vi "Get Paths.vi"(8 "error in":errorcluster, 10 "Naming Data":refnum<class "Naming Data.lvclass">, 11 "Namer With Shared Approved File in":refnum<class "Namer With Shared Approved File.lvclass">) -> (0 "error out":errorcluster, 1 "Received Path":path, 2 "Approved Path":path, 3 "Namer With Shared Approved File out":refnum<class "Namer With Shared Approved File.lvclass">)   [LabVIEW 2020, in "Approval Tests.lvlib" / "Namer With Shared Approved File.lvclass"]
uses:
  Namer With Shared Approved File.lvclass
  Naming Data/Naming Data.lvclass
  Namer With Shared Approved File.lvclass/Namer With Shared Approved File.ctl
  Namer Decorator/Namer Decorator.lvclass
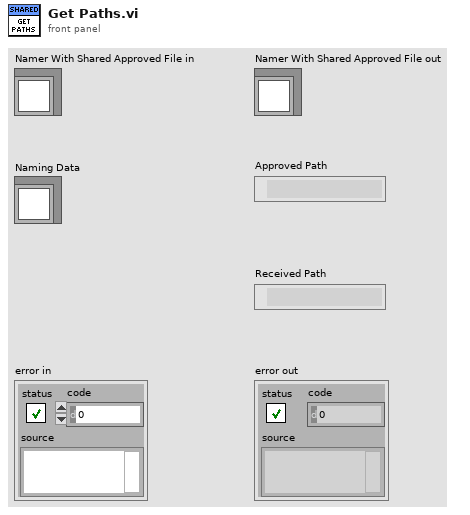
[diagram p1: front panel]
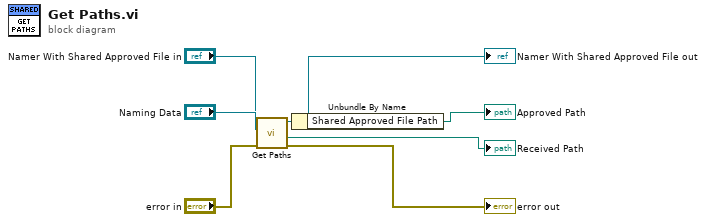
[diagram p0: block diagram]
diagram:
  n1 = call-parent "Get Paths.vi"("error in"="error in", "Naming Data"="Naming Data", "Namer Decorator in"="Namer With Shared Approved File in") -> ("error out"=→"error out":errorcluster, "Received Path"=→"Received Path":path, "Namer Decorator out"=w2:refnum<class "Namer With Shared Approved File.lvclass">)  [unwired: 5 in, 1 out]
  "Namer With Shared Approved File out" <- w2
  n2 = Unbundle By Name(w2) -> ("Shared Approved File Path"=→"Approved Path":path)
